vi "Destroy Processors.vi"(8 "error in (no error)":errorcluster, 11 "ImagePipeline in":refnum<class "ImagePipeline.lvclass">) -> (0 "error out":errorcluster, 3 "ImagePipeline out":refnum<class "ImagePipeline.lvclass">)   [LabVIEW 2020, in "ImagePipeline.lvlib" / "ImagePipeline.lvclass"]
uses:
  ImagePipeline.lvclass
  ImagePipeline.lvclass/ImagePipeline.ctl
  <vilib>/ActorFramework/Message Enqueuer/Message Enqueuer.lvclass/Message Enqueuer.ctl
  <vilib>/ActorFramework/Message Enqueuer/Enqueue.vi
  <vilib>/ActorFramework/Stop Msg/Stop Msg.lvclass
  C:/Program Files/National Instruments/LabVIEW 2020/vi.lib/ActorFramework/Message/Message.lvclass
  <vilib>/ActorFramework/Message Priority Queue/Priority Enqueue.vi
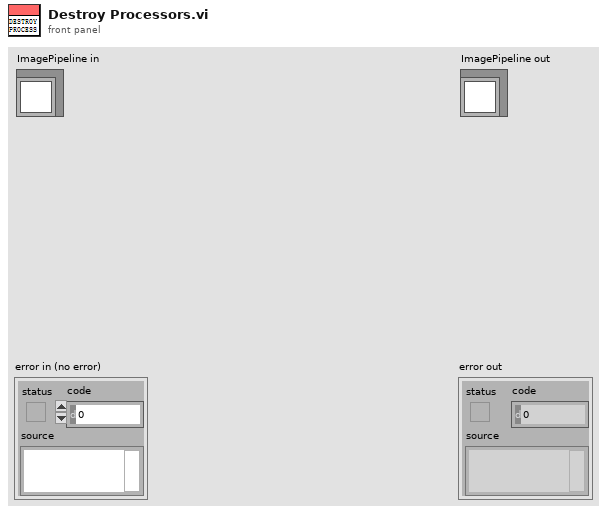
[diagram p1: front panel]
types:
  T1 = map{string, refnum<class "Message Enqueuer.lvclass">}
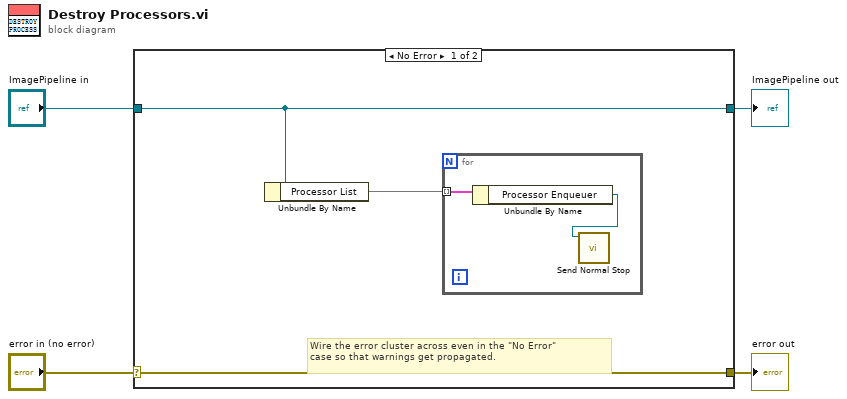
[diagram p0: block diagram]
diagram:
  n1 = case shown="No Error" "error in (no error)" {
    selector: "error in (no error)" -> [w7 w11]
    tunnel: [w7 w11] -> w3
    tunnel: [w6 w10] -> w1
    tunnel: "ImagePipeline in" -> [w6 w10]
    frame No Error {
      # "Wire the error cluster across even in the \"No Error\"\ncase so that warnings get propagated."
      n2 = Unbundle By Name(w6) -> ("Processor List"=w5:T1)
      n3 = for {
        tunnel: w5 -> [w9] mode=indexing
        n4 = Unbundle By Name(w9) -> ("Processor Enqueuer"=w8:refnum<class "Message Enqueuer.lvclass">)
        n5 = call <vilib>:"Send Normal Stop.vi"("Message Enqueuer"=w8) -> ()  [unwired: 10 in, 1 out]
      }
    }
    frame Error {
    }
  }
  "error out" <- w3
  "ImagePipeline out" <- w1
